vi "Set Pin Status.vi"(0 "Cypress in":refnum<class "Cypress.lvclass">, 5 "Port":dbl, 7 "Pin":dbl, 9 "Value":bool, 11 "error in (no error)":errorcluster) -> (4 "Cypress out":refnum<class "Cypress.lvclass">, 15 "error out":errorcluster)   [LabVIEW 2020, in "Cypress.lvclass"]
doc: "Método heredado del padre con un override"
uses:
  Cypress.lvclass
  230bd13b-0866-4034-bcda-73eb21664eb6.vi
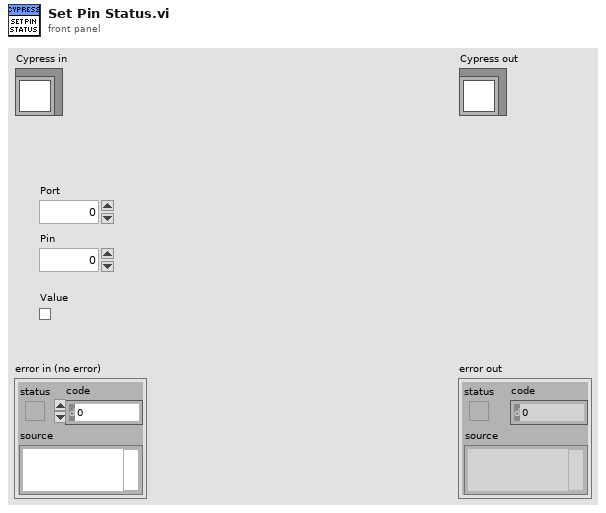
[diagram p1: front panel]
types:
  T1 = typedef "Serial device.lvclass/Brand combobox.ctl" = string
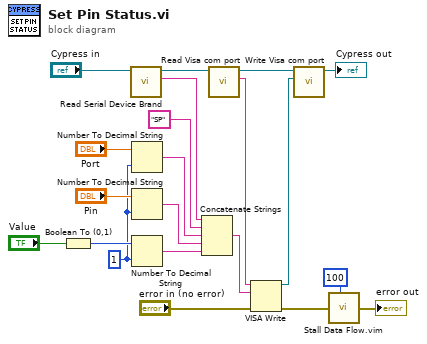
[diagram p0: block diagram]
diagram:
  w1 = i16 1 ("width (-)")
  n1 = Boolean To (0,1)(Boolean="Value") -> (0, 1=w9:i16)
  n2 = call-dynamic "Read Serial Device Brand.vi"("Serial device in"="Cypress in") -> ("Serial Device Brand"=w8:T1, "Serial device out"=w21:refnum<class "Cypress.lvclass">)  [unwired: 8 in, 1 out]
  n3 = Number To Decimal String(number="Port", width (-)=w1) -> (decimal integer string=w4:string)
  n4 = Number To Decimal String(number="Pin", width (-)=w1) -> (decimal integer string=w3:string)
  n5 = Number To Decimal String(number=w9, width (-)=w1) -> (decimal integer string=w2:string)
  n6 = Concatenate Strings(w8, "SP" ("string"), w4, w3, w2) -> (w6:string)
  n7 = call-dynamic "Read Visa com port.vi"("Serial device in"=w21) -> ("Visa com port"=w7:string, "Serial device out"=w20:refnum<class "Cypress.lvclass">)  [unwired: 8 in, 1 out]
  n8 = VISA Write(VISA resource name=w7, write buffer=w6, error in (no error)="error in (no error)") -> (VISA resource name out=w5:refnum<visa-resource-name>, error out=w14:errorcluster)  [unwired: 1 out]
  n9 = call-dynamic "Write Visa com port.vi"("Visa com port"=w5, "Serial device in"=w20) -> ("Serial device out"=→"Cypress out":refnum<class "Cypress.lvclass">)  [unwired: 8 in, 1 out]
  n10 = call "Stall Data Flow.vim"("value in"=w14, "milliseconds to wait"=u32 100) -> ("value out"=→"error out":errorcluster)  [unwired: 1 out]
